vi "Write.vi"(8 "error in (no error)":errorcluster, 10 "Digital Output":bool, 11 "Digital Output in":refnum<class "Digital Output.lvclass">) -> (0 "error out":errorcluster)   [LabVIEW 2021, in "Digital Output.lvclass"]
uses:
  Digital Output.lvclass
  Digital Output.lvclass/Digital Output.ctl
  <vilib>/DAQmx/write.llb/DAQmx Write (Digital Bool 1Line 1Point).vi
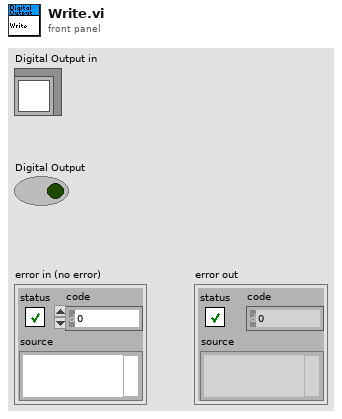
[diagram p1: front panel]
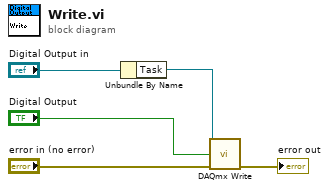
[diagram p0: block diagram]
diagram:
  n1 = Unbundle By Name("Digital Output in") -> ("Task"=w5:refnum<k21>)
  n2 = call-poly <vilib>:"DAQmx Write.vi"("task/channels in"=w5, "data"="Digital Output", "error in"="error in (no error)") -> ("error out"=→"error out":errorcluster)  [unwired: 10 in, 2 out]
